vi "App - analyze RUS V6.vi"() -> ()   [LabVIEW 2021] (continued)
 "lorentzian"={"A (VHz)"=0.0, "ω (Hz)"=0.0, "Γ (Hz)"=0.0, "φ (rad)"=0.0, "Q"=0.0, "Norm  Ampl"=0.0, "z∞ (V)"=0.0+0.0i, "4corners"={"z (-pi/2)"=0.0+0.0i, "z(inf)"=0.0+0.0i, "z (pi/2)"=0.0+0.0i, "z center"=0.0+0.0i, "z(0)"=0.0+0.0i, "radius"=0.0}}, "timestamp(min)"=1596.8000000044703, "timestamp"=timestamp(3493823629 s since 1904-01-01), "Magn Field(T)"=0.0}, {"temperature"=41.326, "lorentzian"={"A (VHz)"=0.0, "ω (Hz)"=0.0, "Γ (Hz)"=0.0, "φ (rad)"=0.0, "Q"=0.0, "Norm  Ampl"=0.0, "z∞ (V)"=0.0+0.0i, "4corners"={"z (-pi/2)"=0.0+0.0i, "z(inf)"=0.0+0.0i, "z (pi/2)"=0.0+0.0i, "z center"=0.0+0.0i, "z(0)"=0.0+0.0i, "radius"=0.0}}, "timestamp(min)"=1598.1166666671634, "timestamp"=timestamp(3493823708 s since 1904-01-01), "Magn Field(T)"=0.0}, {"temperature"=41.255, "lorentzian"={"A (VHz)"=0.0, "ω (Hz)"=0.0, "Γ (Hz)"=0.0, "φ (rad)"=0.0, "Q"=0.0, "Norm  Ampl"=0.0, "z∞ (V)"=0.0+0.0i, "4corners"={"z (-pi/2)"=0.0+0.0i, "z(inf)"=0.0+0.0i, "z (pi/2)"=0.0+0.0i, "z center"=0.0+0.0i, "z(0)"=0.0+0.0i, "radius"=0.0}}, "timestamp(min)"=1599.433333337307, "timestamp"=timestamp(3493823787 s since 1904-01-01), "Magn Field(T)"=0.0}, {"temperature"=41.174, "lorentzian"={"A (VHz)"=0.0, "ω (Hz)"=0.0, "Γ (Hz)"=0.0, "φ (rad)"=0.0, "Q"=0.0, "Norm  Ampl"=0.0, "z∞ (V)"=0.0+0.0i, "4corners"={"z (-pi/2)"=0.0+0.0i, "z(inf)"=0.0+0.0i, "z (pi/2)"=0.0+0.0i, "z center"=0.0+0.0i, "z(0)"=0.0+0.0i, "radius"=0.0}}, "timestamp(min)"=1600.7666666656733, "timestamp"=timestamp(3493823867 s since 1904-01-01), "Magn Field(T)"=0.0}, {"temperature"=41.098, "lorentzian"={"A (VHz)"=0.0, "ω (Hz)"=0.0, "Γ (Hz)"=0.0, "φ (rad)"=0.0, "Q"=0.0, "Norm  Ampl"=0.0, "z∞ (V)"=0.0+0.0i, "4corners"={"z (-pi/2)"=0.0+0.0i, "z(inf)"=0.0+0.0i, "z (pi/2)"=0.0+0.0i, "z center"=0.0+0.0i, "z(0)"=0.0+0.0i, "radius"=0.0}}, "timestamp(min)"=1602.0833333358169, "timestamp"=timestamp(3493823946 s since 1904-01-01), "Magn Field(T)"=0.0}, {"temperature"=41.017, "lorentzian"={"A (VHz)"=0.0, "ω (Hz)"=0.0, "Γ (Hz)"=0.0, "φ (rad)"=0.0, "Q"=0.0, "Norm  Ampl"=0.0, "z∞ (V)"=0.0+0.0i, "4corners"={"z (-pi/2)"=0.0+0.0i, "z(inf)"=0.0+0.0i, "z (pi/2)"=0.0+0.0i, "z center"=0.0+0.0i, "z(0)"=0.0+0.0i, "radius"=0.0}}, "timestamp(min)"=1603.3999999985099, "timestamp"=timestamp(3493824025 s since 1904-01-01), "Magn Field(T)"=0.0}, {"temperature"=40.94, "lorentzian"={"A (VHz)"=0.0, "ω (Hz)"=0.0, "Γ (Hz)"=0.0, "φ (rad)"=0.0, "Q"=0.0, "Norm  Ampl"=0.0, "z∞ (V)"=0.0+0.0i, "4corners"={"z (-pi/2)"=0.0+0.0i, "z(inf)"=0.0+0.0i, "z (pi/2)"=0.0+0.0i, "z center"=0.0+0.0i, "z(0)"=0.0+0.0i, "radius"=0.0}}, "timestamp(min)"=1604.7333333343267, "timestamp"=timestamp(3493824105 s since 1904-01-01), "Magn Field(T)"=0.0}, {"temperature"=40.861, "lorentzian"={"A (VHz)"=0.0, "ω (Hz)"=0.0, "Γ (Hz)"=0.0, "φ (rad)"=0.0, "Q"=0.0, "Norm  Ampl"=0.0, "z∞ (V)"=0.0+0.0i, "4corners"={"z (-pi/2)"=0.0+0.0i, "z(inf)"=0.0+0.0i, "z (pi/2)"=0.0+0.0i, "z center"=0.0+0.0i, "z(0)"=0.0+0.0i, "radius"=0.0}}, "timestamp(min)"=1606.0500000044703, "timestamp"=timestamp(3493824184 s since 1904-01-01), "Magn Field(T)"=0.0}, {"temperature"=40.779, "lorentzian"={"A (VHz)"=0.0, "ω (Hz)"=0.0, "Γ (Hz)"=0.0, "φ (rad)"=0.0, "Q"=0.0, "Norm  Ampl"=0.0, "z∞ (V)"=0.0+0.0i, "4corners"={"z (-pi/2)"=0.0+0.0i, "z(inf)"=0.0+0.0i, "z (pi/2)"=0.0+0.0i, "z center"=0.0+0.0i, "z(0)"=0.0+0.0i, "radius"=0.0}}, "timestamp(min)"=1607.3833333328366, "timestamp"=timestamp(3493824264 s since 1904-01-01), "Magn Field(T)"=0.0}, {"temperature"=40.702, "lorentzian"={"A (VHz)"=0.0, "ω (Hz)"=0.0, "Γ (Hz)"=0.0, "φ (rad)"=0.0, "Q"=0.0, "Norm  Ampl"=0.0, "z∞ (V)"=0.0+0.0i, "4corners"={"z (-pi/2)"=0.0+0.0i, "z(inf)"=0.0+0.0i, "z (pi/2)"=0.0+0.0i, "z center"=0.0+0.0i, "z(0)"=0.0+0.0i, "radius"=0.0}}, "timestamp(min)"=1608.7000000029802, "timestamp"=timestamp(3493824343 s since 1904-01-01), "Magn Field(T)"=0.0}, {"temperature"=40.621, "lorentzian"={"A (VHz)"=0.0, "ω (Hz)"=0.0, "Γ (Hz)"=0.0, "φ (rad)"=0.0, "Q"=0.0, "Norm  Ampl"=0.0, "z∞ (V)"=0.0+0.0i, "4corners"={"z (-pi/2)"=0.0+0.0i, "z(inf)"=0.0+0.0i, "z (pi/2)"=0.0+0.0i, "z center"=0.0+0.0i, "z(0)"=0.0+0.0i, "radius"=0.0}}, "timestamp(min)"=1610.0333333313465, "timestamp"=timestamp(3493824423 s since 1904-01-01), "Magn Field(T)"=0.0}, {"temperature"=40.542, "lorentzian"={"A (VHz)"=0.0, "ω (Hz)"=0.0, "Γ (Hz)"=0.0, "φ (rad)"=0.0, "Q"=0.0, "Norm  Ampl"=0.0, "z∞ (V)"=0.0+0.0i, "4corners"={"z (-pi/2)"=0.0+0.0i, "z(inf)"=0.0+0.0i, "z (pi/2)"=0.0+0.0i, "z center"=0.0+0.0i, "z(0)"=0.0+0.0i, "radius"=0.0}}, "timestamp(min)"=1611.3500000014901, "timestamp"=timestamp(3493824502 s since 1904-01-01), "Magn Field(T)"=0.0}, {"temperature"=40.463, "lorentzian"={"A (VHz)"=0.0, "ω (Hz)"=0.0, "Γ (Hz)"=0.0, "φ (rad)"=0.0, "Q"=0.0, "Norm  Ampl"=0.0, "z∞ (V)"=0.0+0.0i, "4corners"={"z (-pi/2)"=0.0+0.0i, "z(inf)"=0.0+0.0i, "z (pi/2)"=0.0+0.0i, "z center"=0.0+0.0i, "z(0)"=0.0+0.0i, "radius"=0.0}}, "timestamp(min)"=1612.683333337307, "timestamp"=timestamp(3493824582 s since 1904-01-01), "Magn Field(T)"=0.0}, {"temperature"=40.383, "lorentzian"={"A (VHz)"=0.0, "ω (Hz)"=0.0, "Γ (Hz)"=0.0, "φ (rad)"=0.0, "Q"=0.0, "Norm  Ampl"=0.0, "z∞ (V)"=0.0+0.0i, "4corners"={"z (-pi/2)"=0.0+0.0i, "z(inf)"=0.0+0.0i, "z (pi/2)"=0.0+0.0i, "z center"=0.0+0.0i, "z(0)"=0.0+0.0i, "radius"=0.0}}, "timestamp(min)"=1614.0, "timestamp"=timestamp(3493824661 s since 1904-01-01), "Magn Field(T)"=0.0}, {"temperature"=40.311, "lorentzian"={"A (VHz)"=0.0, "ω (Hz)"=0.0, "Γ (Hz)"=0.0, "φ (rad)"=0.0, "Q"=0.0, "Norm  Ampl"=0.0, "z∞ (V)"=0.0+0.0i, "4corners"={"z (-pi/2)"=0.0+0.0i, "z(inf)"=0.0+0.0i, "z (pi/2)"=0.0+0.0i, "z center"=0.0+0.0i, "z(0)"=0.0+0.0i, "radius"=0.0}}, "timestamp(min)"=1615.3333333358169, "timestamp"=timestamp(3493824741 s since 1904-01-01), "Magn Field(T)"=0.0}, {"temperature"=40.223, "lorentzian"={"A (VHz)"=0.0, "ω (Hz)"=0.0, "Γ (Hz)"=0.0, "φ (rad)"=0.0, "Q"=0.0, "Norm  Ampl"=0.0, "z∞ (V)"=0.0+0.0i, "4corners"={"z (-pi/2)"=0.0+0.0i, "z(inf)"=0.0+0.0i, "z (pi/2)"=0.0+0.0i, "z center"=0.0+0.0i, "z(0)"=0.0+0.0i, "radius"=0.0}}, "timestamp(min)"=1616.6499999985099, "timestamp"=timestamp(3493824820 s since 1904-01-01), "Magn Field(T)"=0.0}, {"temperature"=40.145, "lorentzian"={"A (VHz)"=0.0, "ω (Hz)"=0.0, "Γ (Hz)"=0.0, "φ (rad)"=0.0, "Q"=0.0, "Norm  Ampl"=0.0, "z∞ (V)"=0.0+0.0i, "4corners"={"z (-pi/2)"=0.0+0.0i, "z(inf)"=0.0+0.0i, "z (pi/2)"=0.0+0.0i, "z center"=0.0+0.0i, "z(0)"=0.0+0.0i, "radius"=0.0}}, "timestamp(min)"=1617.9666666686535, "timestamp"=timestamp(3493824899 s since 1904-01-01), "Magn Field(T)"=0.0}, {"temperature"=40.07, "lorentzian"={"A (VHz)"=0.0, "ω (Hz)"=0.0, "Γ (Hz)"=0.0, "φ (rad)"=0.0, "Q"=0.0, "Norm  Ampl"=0.0, "z∞ (V)"=0.0+0.0i, "4corners"={"z (-pi/2)"=0.0+0.0i, "z(inf)"=0.0+0.0i, "z (pi/2)"=0.0+0.0i, "z center"=0.0+0.0i, "z(0)"=0.0+0.0i, "radius"=0.0}}, "timestamp(min)"=1619.3000000044703, "timestamp"=timestamp(3493824979 s since 1904-01-01), "Magn Field(T)"=0.0}, {"temperature"=39.984, "lorentzian"={"A (VHz)"=0.0, "ω (Hz)"=0.0, "Γ (Hz)"=0.0, "φ (rad)"=0.0, "Q"=0.0, "Norm  Ampl"=0.0, "z∞ (V)"=0.0+0.0i, "4corners"={"z (-pi/2)"=0.0+0.0i, "z(inf)"=0.0+0.0i, "z (pi/2)"=0.0+0.0i, "z center"=0.0+0.0i, "z(0)"=0.0+0.0i, "radius"=0.0}}, "timestamp(min)"=1620.6166666671634, "timestamp"=timestamp(3493825058 s since 1904-01-01), "Magn Field(T)"=0.0}, {"temperature"=39.905, "lorentzian"={"A (VHz)"=0.0, "ω (Hz)"=0.0, "Γ (Hz)"=0.0, "φ (rad)"=0.0, "Q"=0.0, "Norm  Ampl"=0.0, "z∞ (V)"=0.0+0.0i, "4corners"={"z (-pi/2)"=0.0+0.0i, "z(inf)"=0.0+0.0i, "z (pi/2)"=0.0+0.0i, "z center"=0.0+0.0i, "z(0)"=0.0+0.0i, "radius"=0.0}}, "timestamp(min)"=1621.9500000029802, "timestamp"=timestamp(3493825138 s since 1904-01-01), "Magn Field(T)"=0.0}, {"temperature"=39.827, "lorentzian"={"A (VHz)"=0.0, "ω (Hz)"=0.0, "Γ (Hz)"=0.0, "φ (rad)"=0.0, "Q"=0.0, "Norm  Ampl"=0.0, "z∞ (V)"=0.0+0.0i, "4corners"={"z (-pi/2)"=0.0+0.0i, "z(inf)"=0.0+0.0i, "z (pi/2)"=0.0+0.0i, "z center"=0.0+0.0i, "z(0)"=0.0+0.0i, "radius"=0.0}}, "timestamp(min)"=1623.2666666656733, "timestamp"=timestamp(3493825217 s since 1904-01-01), "Magn Field(T)"=0.0}, {"temperature"=39.744, "lorentzian"={"A (VHz)"=0.0, "ω (Hz)"=0.0, "Γ (Hz)"=0.0, "φ (rad)"=0.0, "Q"=0.0, "Norm  Ampl"=0.0, "z∞ (V)"=0.0+0.0i, "4corners"={"z (-pi/2)"=0.0+0.0i, "z(inf)"=0.0+0.0i, "z (pi/2)"=0.0+0.0i, "z center"=0.0+0.0i, "z(0)"=0.0+0.0i, "radius"=0.0}}, "timestamp(min)"=1624.5833333358169, "timestamp"=timestamp(3493825296 s since 1904-01-01), "Magn Field(T)"=0.0}, {"temperature"=39.665, "lorentzian"={"A (VHz)"=0.0, "ω (Hz)"=0.0, "Γ (Hz)"=0.0, "φ (rad)"=0.0, "Q"=0.0, "Norm  Ampl"=0.0, "z∞ (V)"=0.0+0.0i, "4corners"={"z (-pi/2)"=0.0+0.0i, "z(inf)"=0.0+0.0i, "z (pi/2)"=0.0+0.0i, "z center"=0.0+0.0i, "z(0)"=0.0+0.0i, "radius"=0.0}}, "timestamp(min)"=1625.9166666641831, "timestamp"=timestamp(3493825376 s since 1904-01-01), "Magn Field(T)"=0.0}, {"temperature"=39.59, "lorentzian"={"A (VHz)"=0.0, "ω (Hz)"=0.0, "Γ (Hz)"=0.0, "φ (rad)"=0.0, "Q"=0.0, "Norm  Ampl"=0.0, "z∞ (V)"=0.0+0.0i, "4corners"={"z (-pi/2)"=0.0+0.0i, "z(inf)"=0.0+0.0i, "z (pi/2)"=0.0+0.0i, "z center"=0.0+0.0i, "z(0)"=0.0+0.0i, "radius"=0.0}}, "timestamp(min)"=1627.2333333343267, "timestamp"=timestamp(3493825455 s since 1904-01-01), "Magn Field(T)"=0.0}, {"temperature"=39.502, "lorentzian"={"A (VHz)"=0.0, "ω (Hz)"=0.0, "Γ (Hz)"=0.0, "φ (rad)"=0.0, "Q"=0.0, "Norm  Ampl"=0.0, "z∞ (V)"=0.0+0.0i, "4corners"={"z (-pi/2)"=0.0+0.0i, "z(inf)"=0.0+0.0i, "z (pi/2)"=0.0+0.0i, "z center"=0.0+0.0i, "z(0)"=0.0+0.0i, "radius"=0.0}}, "timestamp(min)"=1628.5666666701436, "timestamp"=timestamp(3493825535 s since 1904-01-01), "Magn Field(T)"=0.0}, {"temperature"=39.427, "lorentzian"={"A (VHz)"=0.0, "ω (Hz)"=0.0, "Γ (Hz)"=0.0, "φ (rad)"=0.0, "Q"=0.0, "Norm  Ampl"=0.0, "z∞ (V)"=0.0+0.0i, "4corners"={"z (-pi/2)"=0.0+0.0i, "z(inf)"=0.0+0.0i, "z (pi/2)"=0.0+0.0i, "z center"=0.0+0.0i, "z(0)"=0.0+0.0i, "radius"=0.0}}, "timestamp(min)"=1629.8833333328366, "timestamp"=timestamp(3493825614 s since 1904-01-01), "Magn Field(T)"=0.0}, {"temperature"=39.345, "lorentzian"={"A (VHz)"=0.0, "ω (Hz)"=0.0, "Γ (Hz)"=0.0, "φ (rad)"=0.0, "Q"=0.0, "Norm  Ampl"=0.0, "z∞ (V)"=0.0+0.0i, "4corners"={"z (-pi/2)"=0.0+0.0i, "z(inf)"=0.0+0.0i, "z (pi/2)"=0.0+0.0i, "z center"=0.0+0.0i, "z(0)"=0.0+0.0i, "radius"=0.0}}, "timestamp(min)"=1631.2000000029802, "timestamp"=timestamp(3493825693 s since 1904-01-01), "Magn Field(T)"=0.0}, {"temperature"=39.266, "lorentzian"={"A (VHz)"=0.0, "ω (Hz)"=0.0, "Γ (Hz)"=0.0, "φ (rad)"=0.0, "Q"=0.0, "Norm  Ampl"=0.0, "z∞ (V)"=0.0+0.0i, "4corners"={"z (-pi/2)"=0.0+0.0i, "z(inf)"=0.0+0.0i, "z (pi/2)"=0.0+0.0i, "z center"=0.0+0.0i, "z(0)"=0.0+0.0i, "radius"=0.0}}, "timestamp(min)"=1632.5333333313465, "timestamp"=timestamp(3493825773 s since 1904-01-01), "Magn Field(T)"=0.0}, {"temperature"=39.182, "lorentzian"={"A (VHz)"=0.0, "ω (Hz)"=0.0, "Γ (Hz)"=0.0, "φ (rad)"=0.0, "Q"=0.0, "Norm  Ampl"=0.0, "z∞ (V)"=0.0+0.0i, "4corners"={"z (-pi/2)"=0.0+0.0i, "z(inf)"=0.0+0.0i, "z (pi/2)"=0.0+0.0i, "z center"=0.0+0.0i, "z(0)"=0.0+0.0i, "radius"=0.0}}, "timestamp(min)"=1633.8500000014901, "timestamp"=timestamp(3493825852 s since 1904-01-01), "Magn Field(T)"=0.0}, {"temperature"=39.106, "lorentzian"={"A (VHz)"=0.0, "ω (Hz)"=0.0, "Γ (Hz)"=0.0, "φ (rad)"=0.0, "Q"=0.0, "Norm  Ampl"=0.0, "z∞ (V)"=0.0+0.0i, "4corners"={"z (-pi/2)"=0.0+0.0i, "z(inf)"=0.0+0.0i, "z (pi/2)"=0.0+0.0i, "z center"=0.0+0.0i, "z(0)"=0.0+0.0i, "radius"=0.0}}, "timestamp(min)"=1635.1666666641831, "timestamp"=timestamp(3493825931 s since 1904-01-01), "Magn Field(T)"=0.0}, {"temperature"=39.022, "lorentzian"={"A (VHz)"=0.0, "ω (Hz)"=0.0, "Γ (Hz)"=0.0, "φ (rad)"=0.0, "Q"=0.0, "Norm  Ampl"=0.0, "z∞ (V)"=0.0+0.0i, "4corners"={"z (-pi/2)"=0.0+0.0i, "z(inf)"=0.0+0.0i, "z (pi/2)"=0.0+0.0i, "z center"=0.0+0.0i, "z(0)"=0.0+0.0i, "radius"=0.0}}, "timestamp(min)"=1636.5, "timestamp"=timestamp(3493826011 s since 1904-01-01), "Magn Field(T)"=0.0}, {"temperature"=38.943, "lorentzian"={"A (VHz)"=0.0, "ω (Hz)"=0.0, "Γ (Hz)"=0.0, "φ (rad)"=0.0, "Q"=0.0, "Norm  Ampl"=0.0, "z∞ (V)"=0.0+0.0i, "4corners"={"z (-pi/2)"=0.0+0.0i, "z(inf)"=0.0+0.0i, "z (pi/2)"=0.0+0.0i, "z center"=0.0+0.0i, "z(0)"=0.0+0.0i, "radius"=0.0}}, "timestamp(min)"=1637.8166666701436, "timestamp"=timestamp(3493826090 s since 1904-01-01), "Magn Field(T)"=0.0}, {"temperature"=38.864, "lorentzian"={"A (VHz)"=0.0, "ω (Hz)"=0.0, "Γ (Hz)"=0.0, "φ (rad)"=0.0, "Q"=0.0, "Norm  Ampl"=0.0, "z∞ (V)"=0.0+0.0i, "4corners"={"z (-pi/2)"=0.0+0.0i, "z(inf)"=0.0+0.0i, "z (pi/2)"=0.0+0.0i, "z center"=0.0+0.0i, "z(0)"=0.0+0.0i, "radius"=0.0}}, "timestamp(min)"=1639.1499999985099, "timestamp"=timestamp(3493826170 s since 1904-01-01), "Magn Field(T)"=0.0}, {"temperature"=38.78, "lorentzian"={"A (VHz)"=0.0, "ω (Hz)"=0.0, "Γ (Hz)"=0.0, "φ (rad)"=0.0, "Q"=0.0, "Norm  Ampl"=0.0, "z∞ (V)"=0.0+0.0i, "4corners"={"z (-pi/2)"=0.0+0.0i, "z(inf)"=0.0+0.0i, "z (pi/2)"=0.0+0.0i, "z center"=0.0+0.0i, "z(0)"=0.0+0.0i, "radius"=0.0}}, "timestamp(min)"=1640.4666666686535, "timestamp"=timestamp(3493826249 s since 1904-01-01), "Magn Field(T)"=0.0}, {"temperature"=38.695, "lorentzian"={"A (VHz)"=0.0, "ω (Hz)"=0.0, "Γ (Hz)"=0.0, "φ (rad)"=0.0, "Q"=0.0, "Norm  Ampl"=0.0, "z∞ (V)"=0.0+0.0i, "4corners"={"z (-pi/2)"=0.0+0.0i, "z(inf)"=0.0+0.0i, "z (pi/2)"=0.0+0.0i, "z center"=0.0+0.0i, "z(0)"=0.0+0.0i, "radius"=0.0}}, "timestamp(min)"=1641.8000000044703, "timestamp"=timestamp(3493826329 s since 1904-01-01), "Magn Field(T)"=0.0}, {"temperature"=38.618, "lorentzian"={"A (VHz)"=0.0, "ω (Hz)"=0.0, "Γ (Hz)"=0.0, "φ (rad)"=0.0, "Q"=0.0, "Norm  Ampl"=0.0, "z∞ (V)"=0.0+0.0i, "4corners"={"z (-pi/2)"=0.0+0.0i, "z(inf)"=0.0+0.0i, "z (pi/2)"=0.0+0.0i, "z center"=0.0+0.0i, "z(0)"=0.0+0.0i, "radius"=0.0}}, "timestamp(min)"=1643.1166666671634, "timestamp"=timestamp(3493826408 s since 1904-01-01), "Magn Field(T)"=0.0}, {"temperature"=38.531, "lorentzian"={"A (VHz)"=0.0, "ω (Hz)"=0.0, "Γ (Hz)"=0.0, "φ (rad)"=0.0, "Q"=0.0, "Norm  Ampl"=0.0, "z∞ (V)"=0.0+0.0i, "4corners"={"z (-pi/2)"=0.0+0.0i, "z(inf)"=0.0+0.0i, "z (pi/2)"=0.0+0.0i, "z center"=0.0+0.0i, "z(0)"=0.0+0.0i, "radius"=0.0}}, "timestamp(min)"=1644.433333337307, "timestamp"=timestamp(3493826487 s since 1904-01-01), "Magn Field(T)"=0.0}, {"temperature"=38.455, "lorentzian"={"A (VHz)"=0.0, "ω (Hz)"=0.0, "Γ (Hz)"=0.0, "φ (rad)"=0.0, "Q"=0.0, "Norm  Ampl"=0.0, "z∞ (V)"=0.0+0.0i, "4corners"={"z (-pi/2)"=0.0+0.0i, "z(inf)"=0.0+0.0i, "z (pi/2)"=0.0+0.0i, "z center"=0.0+0.0i, "z(0)"=0.0+0.0i, "radius"=0.0}}, "timestamp(min)"=1645.7666666656733, "timestamp"=timestamp(3493826567 s since 1904-01-01), "Magn Field(T)"=0.0}, {"temperature"=38.37, "lorentzian"={"A (VHz)"=0.0, "ω (Hz)"=0.0, "Γ (Hz)"=0.0, "φ (rad)"=0.0, "Q"=0.0, "Norm  Ampl"=0.0, "z∞ (V)"=0.0+0.0i, "4corners"={"z (-pi/2)"=0.0+0.0i, "z(inf)"=0.0+0.0i, "z (pi/2)"=0.0+0.0i, "z center"=0.0+0.0i, "z(0)"=0.0+0.0i, "radius"=0.0}}, "timestamp(min)"=1647.0833333358169, "timestamp"=timestamp(3493826646 s since 1904-01-01), "Magn Field(T)"=0.0}, {"temperature"=38.286, "lorentzian"={"A (VHz)"=0.0, "ω (Hz)"=0.0, "Γ (Hz)"=0.0, "φ (rad)"=0.0, "Q"=0.0, "Norm  Ampl"=0.0, "z∞ (V)"=0.0+0.0i, "4corners"={"z (-pi/2)"=0.0+0.0i, "z(inf)"=0.0+0.0i, "z (pi/2)"=0.0+0.0i, "z center"=0.0+0.0i, "z(0)"=0.0+0.0i, "radius"=0.0}}, "timestamp(min)"=1648.3999999985099, "timestamp"=timestamp(3493826725 s since 1904-01-01), "Magn Field(T)"=0.0}, {"temperature"=38.203, "lorentzian"={"A (VHz)"=0.0, "ω (Hz)"=0.0, "Γ (Hz)"=0.0, "φ (rad)"=0.0, "Q"=0.0, "Norm  Ampl"=0.0, "z∞ (V)"=0.0+0.0i, "4corners"={"z (-pi/2)"=0.0+0.0i, "z(inf)"=0.0+0.0i, "z (pi/2)"=0.0+0.0i, "z center"=0.0+0.0i, "z(0)"=0.0+0.0i, "radius"=0.0}}, "timestamp(min)"=1649.7333333343267, "timestamp"=timestamp(3493826805 s since 1904-01-01), "Magn Field(T)"=0.0}, {"temperature"=38.122, "lorentzian"={"A (VHz)"=0.0, "ω (Hz)"=0.0, "Γ (Hz)"=0.0, "φ (rad)"=0.0, "Q"=0.0, "Norm  Ampl"=0.0, "z∞ (V)"=0.0+0.0i, "4corners"={"z (-pi/2)"=0.0+0.0i, "z(inf)"=0.0+0.0i, "z (pi/2)"=0.0+0.0i, "z center"=0.0+0.0i, "z(0)"=0.0+0.0i, "radius"=0.0}}, "timestamp(min)"=1651.0500000044703, "timestamp"=timestamp(3493826884 s since 1904-01-01), "Magn Field(T)"=0.0}, {"temperature"=38.042, "lorentzian"={"A (VHz)"=0.0, "ω (Hz)"=0.0, "Γ (Hz)"=0.0, "φ (rad)"=0.0, "Q"=0.0, "Norm  Ampl"=0.0, "z∞ (V)"=0.0+0.0i, "4corners"={"z (-pi/2)"=0.0+0.0i, "z(inf)"=0.0+0.0i, "z (pi/2)"=0.0+0.0i, "z center"=0.0+0.0i, "z(0)"=0.0+0.0i, "radius"=0.0}}, "timestamp(min)"=1652.3833333328366, "timestamp"=timestamp(3493826964 s since 1904-01-01), "Magn Field(T)"=0.0}, {"temperature"=37.958, "lorentzian"={"A (VHz)"=0.0, "ω (Hz)"=0.0, "Γ (Hz)"=0.0, "φ (rad)"=0.0, "Q"=0.0, "Norm  Ampl"=0.0, "z∞ (V)"=0.0+0.0i, "4corners"={"z (-pi/2)"=0.0+0.0i, "z(inf)"=0.0+0.0i, "z (pi/2)"=0.0+0.0i, "z center"=0.0+0.0i, "z(0)"=0.0+0.0i, "radius"=0.0}}, "timestamp(min)"=1653.7000000029802, "timestamp"=timestamp(3493827043 s since 1904-01-01), "Magn Field(T)"=0.0}, {"temperature"=37.876, "lorentzian"={"A (VHz)"=0.0, "ω (Hz)"=0.0, "Γ (Hz)"=0.0, "φ (rad)"=0.0, "Q"=0.0, "Norm  Ampl"=0.0, "z∞ (V)"=0.0+0.0i, "4corners"={"z (-pi/2)"=0.0+0.0i, "z(inf)"=0.0+0.0i, "z (pi/2)"=0.0+0.0i, "z center"=0.0+0.0i, "z(0)"=0.0+0.0i, "radius"=0.0}}, "timestamp(min)"=1655.0166666656733, "timestamp"=timestamp(3493827122 s since 1904-01-01), "Magn Field(T)"=0.0}, {"temperature"=37.797, "lorentzian"={"A (VHz)"=0.0, "ω (Hz)"=0.0, "Γ (Hz)"=0.0, "φ (rad)"=0.0, "Q"=0.0, "Norm  Ampl"=0.0, "z∞ (V)"=0.0+0.0i, "4corners"={"z (-pi/2)"=0.0+0.0i, "z(inf)"=0.0+0.0i, "z (pi/2)"=0.0+0.0i, "z center"=0.0+0.0i, "z(0)"=0.0+0.0i, "radius"=0.0}}, "timestamp(min)"=1656.3500000014901, "timestamp"=timestamp(3493827202 s since 1904-01-01), "Magn Field(T)"=0.0}, {"temperature"=37.711, "lorentzian"={"A (VHz)"=0.0, "ω (Hz)"=0.0, "Γ (Hz)"=0.0, "φ (rad)"=0.0, "Q"=0.0, "Norm  Ampl"=0.0, "z∞ (V)"=0.0+0.0i, "4corners"={"z (-pi/2)"=0.0+0.0i, "z(inf)"=0.0+0.0i, "z (pi/2)"=0.0+0.0i, "z center"=0.0+0.0i, "z(0)"=0.0+0.0i, "radius"=0.0}}, "timestamp(min)"=1657.6666666641831, "timestamp"=timestamp(3493827281 s since 1904-01-01), "Magn Field(T)"=0.0}, {"temperature"=37.627, "lorentzian"={"A (VHz)"=0.0, "ω (Hz)"=0.0, "Γ (Hz)"=0.0, "φ (rad)"=0.0, "Q"=0.0, "Norm  Ampl"=0.0, "z∞ (V)"=0.0+0.0i, "4corners"={"z (-pi/2)"=0.0+0.0i, "z(inf)"=0.0+0.0i, "z (pi/2)"=0.0+0.0i, "z center"=0.0+0.0i, "z(0)"=0.0+0.0i, "radius"=0.0}}, "timestamp(min)"=1658.9833333343267, "timestamp"=timestamp(3493827360 s since 1904-01-01), "Magn Field(T)"=0.0}, {"temperature"=37.544, "lorentzian"={"A (VHz)"=0.0, "ω (Hz)"=0.0, "Γ (Hz)"=0.0, "φ (rad)"=0.0, "Q"=0.0, "Norm  Ampl"=0.0, "z∞ (V)"=0.0+0.0i, "4corners"={"z (-pi/2)"=0.0+0.0i, "z(inf)"=0.0+0.0i, "z (pi/2)"=0.0+0.0i, "z center"=0.0+0.0i, "z(0)"=0.0+0.0i, "radius"=0.0}}, "timestamp(min)"=1660.3166666701436, "timestamp"=timestamp(3493827440 s since 1904-01-01), "Magn Field(T)"=0.0}, {"temperature"=37.459, "lorentzian"={"A (VHz)"=0.0, "ω (Hz)"=0.0, "Γ (Hz)"=0.0, "φ (rad)"=0.0, "Q"=0.0, "Norm  Ampl"=0.0, "z∞ (V)"=0.0+0.0i, "4corners"={"z (-pi/2)"=0.0+0.0i, "z(inf)"=0.0+0.0i, "z (pi/2)"=0.0+0.0i, "z center"=0.0+0.0i, "z(0)"=0.0+0.0i, "radius"=0.0}}, "timestamp(min)"=1661.6333333328366, "timestamp"=timestamp(3493827519 s since 1904-01-01), "Magn Field(T)"=0.0}, {"temperature"=37.378, "lorentzian"={"A (VHz)"=0.0, "ω (Hz)"=0.0, "Γ (Hz)"=0.0, "φ (rad)"=0.0, "Q"=0.0, "Norm  Ampl"=0.0, "z∞ (V)"=0.0+0.0i, "4corners"={"z (-pi/2)"=0.0+0.0i, "z(inf)"=0.0+0.0i, "z (pi/2)"=0.0+0.0i, "z center"=0.0+0.0i, "z(0)"=0.0+0.0i, "radius"=0.0}}, "timestamp(min)"=1662.9666666686535, "timestamp"=timestamp(3493827599 s since 1904-01-01), "Magn Field(T)"=0.0}, {"temperature"=37.297, "lorentzian"={"A (VHz)"=0.0, "ω (Hz)"=0.0, "Γ (Hz)"=0.0, "φ (rad)"=0.0, "Q"=0.0, "Norm  Ampl"=0.0, "z∞ (V)"=0.0+0.0i, "4corners"={"z (-pi/2)"=0.0+0.0i, "z(inf)"=0.0+0.0i, "z (pi/2)"=0.0+0.0i, "z center"=0.0+0.0i, "z(0)"=0.0+0.0i, "radius"=0.0}}, "timestamp(min)"=1664.2833333313465, "timestamp"=timestamp(3493827678 s since 1904-01-01), "Magn Field(T)"=0.0}, {"temperature"=37.206, "lorentzian"={"A (VHz)"=0.0, "ω (Hz)"=0.0, "Γ (Hz)"=0.0, "φ (rad)"=0.0, "Q"=0.0, "Norm  Ampl"=0.0, "z∞ (V)"=0.0+0.0i, "4corners"={"z (-pi/2)"=0.0+0.0i, "z(inf)"=0.0+0.0i, "z (pi/2)"=0.0+0.0i, "z center"=0.0+0.0i, "z(0)"=0.0+0.0i, "radius"=0.0}}, "timestamp(min)"=1665.6000000014901, "timestamp"=timestamp(3493827757 s since 1904-01-01), "Magn Field(T)"=0.0}, {"temperature"=37.129, "lorentzian"={"A (VHz)"=0.0, "ω (Hz)"=0.0, "Γ (Hz)"=0.0, "φ (rad)"=0.0, "Q"=0.0, "Norm  Ampl"=0.0, "z∞ (V)"=0.0+0.0i, "4corners"={"z (-pi/2)"=0.0+0.0i, "z(inf)"=0.0+0.0i, "z (pi/2)"=0.0+0.0i, "z center"=0.0+0.0i, "z(0)"=0.0+0.0i, "radius"=0.0}}, "timestamp(min)"=1666.933333337307, "timestamp"=timestamp(3493827837 s since 1904-01-01), "Magn Field(T)"=0.0}, {"temperature"=37.038, "lorentzian"={"A (VHz)"=0.0, "ω (Hz)"=0.0, "Γ (Hz)"=0.0, "φ (rad)"=0.0, "Q"=0.0, "Norm  Ampl"=0.0, "z∞ (V)"=0.0+0.0i, "4corners"={"z (-pi/2)"=0.0+0.0i, "z(inf)"=0.0+0.0i, "z (pi/2)"=0.0+0.0i, "z center"=0.0+0.0i, "z(0)"=0.0+0.0i, "radius"=0.0}}, "timestamp(min)"=1668.25, "timestamp"=timestamp(3493827916 s since 1904-01-01), "Magn Field(T)"=0.0}, {"temperature"=36.964, "lorentzian"={"A (VHz)"=0.0, "ω (Hz)"=0.0, "Γ (Hz)"=0.0, "φ (rad)"=0.0, "Q"=0.0, "Norm  Ampl"=0.0, "z∞ (V)"=0.0+0.0i, "4corners"={"z (-pi/2)"=0.0+0.0i, "z(inf)"=0.0+0.0i, "z (pi/2)"=0.0+0.0i, "z center"=0.0+0.0i, "z(0)"=0.0+0.0i, "radius"=0.0}}, "timestamp(min)"=1669.5666666701436, "timestamp"=timestamp(3493827995 s since 1904-01-01), "Magn Field(T)"=0.0}, {"temperature"=36.875, "lorentzian"={"A (VHz)"=0.0, "ω (Hz)"=0.0, "Γ (Hz)"=0.0, "φ (rad)"=0.0, "Q"=0.0, "Norm  Ampl"=0.0, "z∞ (V)"=0.0+0.0i, "4corners"={"z (-pi/2)"=0.0+0.0i, "z(inf)"=0.0+0.0i, "z (pi/2)"=0.0+0.0i, "z center"=0.0+0.0i, "z(0)"=0.0+0.0i, "radius"=0.0}}, "timestamp(min)"=1670.8999999985099, "timestamp"=timestamp(3493828075 s since 1904-01-01), "Magn Field(T)"=0.0}, {"temperature"=36.787, "lorentzian"={"A (VHz)"=0.0, "ω (Hz)"=0.0, "Γ (Hz)"=0.0, "φ (rad)"=0.0, "Q"=0.0, "Norm  Ampl"=0.0, "z∞ (V)"=0.0+0.0i, "4corners"={"z (-pi/2)"=0.0+0.0i, "z(inf)"=0.0+0.0i, "z (pi/2)"=0.0+0.0i, "z center"=0.0+0.0i, "z(0)"=0.0+0.0i, "radius"=0.0}}, "timestamp(min)"=1672.2166666686535, "timestamp"=timestamp(3493828154 s since 1904-01-01), "Magn Field(T)"=0.0}, {"temperature"=36.71, "lorentzian"={"A (VHz)"=0.0, "ω (Hz)"=0.0, "Γ (Hz)"=0.0, "φ (rad)"=0.0, "Q"=0.0, "Norm  Ampl"=0.0, "z∞ (V)"=0.0+0.0i, "4corners"={"z (-pi/2)"=0.0+0.0i, "z(inf)"=0.0+0.0i, "z (pi/2)"=0.0+0.0i, "z center"=0.0+0.0i, "z(0)"=0.0+0.0i, "radius"=0.0}}, "timestamp(min)"=1673.5500000044703, "timestamp"=timestamp(3493828234 s since 1904-01-01), "Magn Field(T)"=0.0}, {"temperature"=36.616, "lorentzian"={"A (VHz)"=0.0, "ω (Hz)"=0.0, "Γ (Hz)"=0.0, "φ (rad)"=0.0, "Q"=0.0, "Norm  Ampl"=0.0, "z∞ (V)"=0.0+0.0i, "4corners"={"z (-pi/2)"=0.0+0.0i, "z(inf)"=0.0+0.0i, "z (pi/2)"=0.0+0.0i, "z center"=0.0+0.0i, "z(0)"=0.0+0.0i, "radius"=0.0}}, "timestamp(min)"=1674.8666666671634, "timestamp"=timestamp(3493828313 s since 1904-01-01), "Magn Field(T)"=0.0}, {"temperature"=36.538, "lorentzian"={"A (VHz)"=0.0, "ω (Hz)"=0.0, "Γ (Hz)"=0.0, "φ (rad)"=0.0, "Q"=0.0, "Norm  Ampl"=0.0, "z∞ (V)"=0.0+0.0i, "4corners"={"z (-pi/2)"=0.0+0.0i, "z(inf)"=0.0+0.0i, "z (pi/2)"=0.0+0.0i, "z center"=0.0+0.0i, "z(0)"=0.0+0.0i, "radius"=0.0}}, "timestamp(min)"=1676.183333337307, "timestamp"=timestamp(3493828392 s since 1904-01-01), "Magn Field(T)"=0.0}, {"temperature"=36.457, "lorentzian"={"A (VHz)"=0.0, "ω (Hz)"=0.0, "Γ (Hz)"=0.0, "φ (rad)"=0.0, "Q"=0.0, "Norm  Ampl"=0.0, "z∞ (V)"=0.0+0.0i, "4corners"={"z (-pi/2)"=0.0+0.0i, "z(inf)"=0.0+0.0i, "z (pi/2)"=0.0+0.0i, "z center"=0.0+0.0i, "z(0)"=0.0+0.0i, "radius"=0.0}}, "timestamp(min)"=1677.5166666656733, "timestamp"=timestamp(3493828472 s since 1904-01-01), "Magn Field(T)"=0.0}, {"temperature"=36.365, "lorentzian"={"A (VHz)"=0.0, "ω (Hz)"=0.0, "Γ (Hz)"=0.0, "φ (rad)"=0.0, "Q"=0.0, "Norm  Ampl"=0.0, "z∞ (V)"=0.0+0.0i, "4corners"={"z (-pi/2)"=0.0+0.0i, "z(inf)"=0.0+0.0i, "z (pi/2)"=0.0+0.0i, "z center"=0.0+0.0i, "z(0)"=0.0+0.0i, "radius"=0.0}}, "timestamp(min)"=1678.8333333358169, "timestamp"=timestamp(3493828551 s since 1904-01-01), "Magn Field(T)"=0.0}, {"temperature"=36.288, "lorentzian"={"A (VHz)"=0.0, "ω (Hz)"=0.0, "Γ (Hz)"=0.0, "φ (rad)"=0.0, "Q"=0.0, "Norm  Ampl"=0.0, "z∞ (V)"=0.0+0.0i, "4corners"={"z (-pi/2)"=0.0+0.0i, "z(inf)"=0.0+0.0i, "z (pi/2)"=0.0+0.0i, "z center"=0.0+0.0i, "z(0)"=0.0+0.0i, "radius"=0.0}}, "timestamp(min)"=1680.1666666641831, "timestamp"=timestamp(3493828631 s since 1904-01-01), "Magn Field(T)"=0.0}, {"temperature"=36.202, "lorentzian"={"A (VHz)"=0.0, "ω (Hz)"=0.0, "Γ (Hz)"=0.0, "φ (rad)"=0.0, "Q"=0.0, "Norm  Ampl"=0.0, "z∞ (V)"=0.0+0.0i, "4corners"={"z (-pi/2)"=0.0+0.0i, "z(inf)"=0.0+0.0i, "z (pi/2)"=0.0+0.0i, "z center"=0.0+0.0i, "z(0)"=0.0+0.0i, "radius"=0.0}}, "timestamp(min)"=1681.4833333343267, "timestamp"=timestamp(3493828710 s since 1904-01-01), "Magn Field(T)"=0.0}, {"temperature"=36.116, "lorentzian"={"A (VHz)"=0.0, "ω (Hz)"=0.0, "Γ (Hz)"=0.0, "φ (rad)"=0.0, "Q"=0.0, "Norm  Ampl"=0.0, "z∞ (V)"=0.0+0.0i, "4corners"={"z (-pi/2)"=0.0+0.0i, "z(inf)"=0.0+0.0i, "z (pi/2)"=0.0+0.0i, "z center"=0.0+0.0i, "z(0)"=0.0+0.0i, "radius"=0.0}}, "timestamp(min)"=1682.8000000044703, "timestamp"=timestamp(3493828789 s since 1904-01-01), "Magn Field(T)"=0.0}, {"temperature"=36.028, "lorentzian"={"A (VHz)"=0.0, "ω (Hz)"=0.0, "Γ (Hz)"=0.0, "φ (rad)"=0.0, "Q"=0.0, "Norm  Ampl"=0.0, "z∞ (V)"=0.0+0.0i, "4corners"={"z (-pi/2)"=0.0+0.0i, "z(inf)"=0.0+0.0i, "z (pi/2)"=0.0+0.0i, "z center"=0.0+0.0i, "z(0)"=0.0+0.0i, "radius"=0.0}}, "timestamp(min)"=1684.1333333328366, "timestamp"=timestamp(3493828869 s since 1904-01-01), "Magn Field(T)"=0.0}, {"temperature"=35.946, "lorentzian"={"A (VHz)"=0.0, "ω (Hz)"=0.0, "Γ (Hz)"=0.0, "φ (rad)"=0.0, "Q"=0.0, "Norm  Ampl"=0.0, "z∞ (V)"=0.0+0.0i, "4corners"={"z (-pi/2)"=0.0+0.0i, "z(inf)"=0.0+0.0i, "z (pi/2)"=0.0+0.0i, "z center"=0.0+0.0i, "z(0)"=0.0+0.0i, "radius"=0.0}}, "timestamp(min)"=1685.4500000029802, "timestamp"=timestamp(3493828948 s since 1904-01-01), "Magn Field(T)"=0.0}, {"temperature"=35.859, "lorentzian"={"A (VHz)"=0.0, "ω (Hz)"=0.0, "Γ (Hz)"=0.0, "φ (rad)"=0.0, "Q"=0.0, "Norm  Ampl"=0.0, "z∞ (V)"=0.0+0.0i, "4corners"={"z (-pi/2)"=0.0+0.0i, "z(inf)"=0.0+0.0i, "z (pi/2)"=0.0+0.0i, "z center"=0.0+0.0i, "z(0)"=0.0+0.0i, "radius"=0.0}}, "timestamp(min)"=1686.7666666656733, "timestamp"=timestamp(3493829027 s since 1904-01-01), "Magn Field(T)"=0.0}, {"temperature"=35.776, "lorentzian"={"A (VHz)"=0.0, "ω (Hz)"=0.0, "Γ (Hz)"=0.0, "φ (rad)"=0.0, "Q"=0.0, "Norm  Ampl"=0.0, "z∞ (V)"=0.0+0.0i, "4corners"={"z (-pi/2)"=0.0+0.0i, "z(inf)"=0.0+0.0i, "z (pi/2)"=0.0+0.0i, "z center"=0.0+0.0i, "z(0)"=0.0+0.0i, "radius"=0.0}}, "timestamp(min)"=1688.1000000014901, "timestamp"=timestamp(3493829107 s since 1904-01-01), "Magn Field(T)"=0.0}, {"temperature"=35.691, "lorentzian"={"A (VHz)"=0.0, "ω (Hz)"=0.0, "Γ (Hz)"=0.0, "φ (rad)"=0.0, "Q"=0.0, "Norm  Ampl"=0.0, "z∞ (V)"=0.0+0.0i, "4corners"={"z (-pi/2)"=0.0+0.0i, "z(inf)"=0.0+0.0i, "z (pi/2)"=0.0+0.0i, "z center"=0.0+0.0i, "z(0)"=0.0+0.0i, "radius"=0.0}}, "timestamp(min)"=1689.4166666641831, "timestamp"=timestamp(3493829186 s since 1904-01-01), "Magn Field(T)"=0.0}, {"temperature"=35.608, "lorentzian"={"A (VHz)"=0.0, "ω (Hz)"=0.0, "Γ (Hz)"=0.0, "φ (rad)"=0.0, "Q"=0.0, "Norm  Ampl"=0.0, "z∞ (V)"=0.0+0.0i, "4corners"={"z (-pi/2)"=0.0+0.0i, "z(inf)"=0.0+0.0i, "z (pi/2)"=0.0+0.0i, "z center"=0.0+0.0i, "z(0)"=0.0+0.0i, "radius"=0.0}}, "timestamp(min)"=1690.75, "timestamp"=timestamp(3493829266 s since 1904-01-01), "Magn Field(T)"=0.0}, {"temperature"=35.519, "lorentzian"={"A (VHz)"=0.0, "ω (Hz)"=0.0, "Γ (Hz)"=0.0, "φ (rad)"=0.0, "Q"=0.0, "Norm  Ampl"=0.0, "z∞ (V)"=0.0+0.0i, "4corners"={"z (-pi/2)"=0.0+0.0i, "z(inf)"=0.0+0.0i, "z (pi/2)"=0.0+0.0i, "z center"=0.0+0.0i, "z(0)"=0.0+0.0i, "radius"=0.0}}, "timestamp(min)"=1692.0666666701436, "timestamp"=timestamp(3493829345 s since 1904-01-01), "Magn Field(T)"=0.0}, {"temperature"=35.437, "lorentzian"={"A (VHz)"=0.0, "ω (Hz)"=0.0, "Γ (Hz)"=0.0, "φ (rad)"=0.0, "Q"=0.0, "Norm  Ampl"=0.0, "z∞ (V)"=0.0+0.0i, "4corners"={"z (-pi/2)"=0.0+0.0i, "z(inf)"=0.0+0.0i, "z (pi/2)"=0.0+0.0i, "z center"=0.0+0.0i, "z(0)"=0.0+0.0i, "radius"=0.0}}, "timestamp(min)"=1693.3833333328366, "timestamp"=timestamp(3493829424 s since 1904-01-01), "Magn Field(T)"=0.0}, {"temperature"=35.349, "lorentzian"={"A (VHz)"=0.0, "ω (Hz)"=0.0, "Γ (Hz)"=0.0, "φ (rad)"=0.0, "Q"=0.0, "Norm  Ampl"=0.0, "z∞ (V)"=0.0+0.0i, "4corners"={"z (-pi/2)"=0.0+0.0i, "z(inf)"=0.0+0.0i, "z (pi/2)"=0.0+0.0i, "z center"=0.0+0.0i, "z(0)"=0.0+0.0i, "radius"=0.0}}, "timestamp(min)"=1694.7166666686535, "timestamp"=timestamp(3493829504 s since 1904-01-01), "Magn Field(T)"=0.0}, {"temperature"=35.264, "lorentzian"={"A (VHz)"=0.0, "ω (Hz)"=0.0, "Γ (Hz)"=0.0, "φ (rad)"=0.0, "Q"=0.0, "Norm  Ampl"=0.0, "z∞ (V)"=0.0+0.0i, "4corners"={"z (-pi/2)"=0.0+0.0i, "z(inf)"=0.0+0.0i, "z (pi/2)"=0.0+0.0i, "z center"=0.0+0.0i, "z(0)"=0.0+0.0i, "radius"=0.0}}, "timestamp(min)"=1696.0333333313465, "timestamp"=timestamp(3493829583 s since 1904-01-01), "Magn Field(T)"=0.0}, {"temperature"=35.178, "lorentzian"={"A (VHz)"=0.0, "ω (Hz)"=0.0, "Γ (Hz)"=0.0, "φ (rad)"=0.0, "Q"=0.0, "Norm  Ampl"=0.0, "z∞ (V)"=0.0+0.0i, "4corners"={"z (-pi/2)"=0.0+0.0i, "z(inf)"=0.0+0.0i, "z (pi/2)"=0.0+0.0i, "z center"=0.0+0.0i, "z(0)"=0.0+0.0i, "radius"=0.0}}, "timestamp(min)"=1697.3666666671634, "timestamp"=timestamp(3493829663 s since 1904-01-01), "Magn Field(T)"=0.0}, {"temperature"=35.091, "lorentzian"={"A (VHz)"=0.0, "ω (Hz)"=0.0, "Γ (Hz)"=0.0, "φ (rad)"=0.0, "Q"=0.0, "Norm  Ampl"=0.0, "z∞ (V)"=0.0+0.0i, "4corners"={"z (-pi/2)"=0.0+0.0i, "z(inf)"=0.0+0.0i, "z (pi/2)"=0.0+0.0i, "z center"=0.0+0.0i, "z(0)"=0.0+0.0i, "radius"=0.0}}, "timestamp(min)"=1698.683333337307, "timestamp"=timestamp(3493829742 s since 1904-01-01), "Magn Field(T)"=0.0}, {"temperature"=35.004, "lorentzian"={"A (VHz)"=0.0, "ω (Hz)"=0.0, "Γ (Hz)"=0.0, "φ (rad)"=0.0, "Q"=0.0, "Norm  Ampl"=0.0, "z∞ (V)"=0.0+0.0i, "4corners"={"z (-pi/2)"=0.0+0.0i, "z(inf)"=0.0+0.0i, "z (pi/2)"=0.0+0.0i, "z center"=0.0+0.0i, "z(0)"=0.0+0.0i, "radius"=0.0}}, "timestamp(min)"=1700.0, "timestamp"=timestamp(3493829821 s since 1904-01-01), "Magn Field(T)"=0.0}, {"temperature"=34.918, "lorentzian"={"A (VHz)"=0.0, "ω (Hz)"=0.0, "Γ (Hz)"=0.0, "φ (rad)"=0.0, "Q"=0.0, "Norm  Ampl"=0.0, "z∞ (V)"=0.0+0.0i, "4corners"={"z (-pi/2)"=0.0+0.0i, "z(inf)"=0.0+0.0i, "z (pi/2)"=0.0+0.0i, "z center"=0.0+0.0i, "z(0)"=0.0+0.0i, "radius"=0.0}}, "timestamp(min)"=1701.3333333358169, "timestamp"=timestamp(3493829901 s since 1904-01-01), "Magn Field(T)"=0.0}, {"temperature"=34.836, "lorentzian"={"A (VHz)"=0.0, "ω (Hz)"=0.0, "Γ (Hz)"=0.0, "φ (rad)"=0.0, "Q"=0.0, "Norm  Ampl"=0.0, "z∞ (V)"=0.0+0.0i, "4corners"={"z (-pi/2)"=0.0+0.0i, "z(inf)"=0.0+0.0i, "z (pi/2)"=0.0+0.0i, "z center"=0.0+0.0i, "z(0)"=0.0+0.0i, "radius"=0.0}}, "timestamp(min)"=1702.6499999985099, "timestamp"=timestamp(3493829980 s since 1904-01-01), "Magn Field(T)"=0.0}, {"temperature"=34.745, "lorentzian"={"A (VHz)"=0.0, "ω (Hz)"=0.0, "Γ (Hz)"=0.0, "φ (rad)"=0.0, "Q"=0.0, "Norm  Ampl"=0.0, "z∞ (V)"=0.0+0.0i, "4corners"={"z (-pi/2)"=0.0+0.0i, "z(inf)"=0.0+0.0i, "z (pi/2)"=0.0+0.0i, "z center"=0.0+0.0i, "z(0)"=0.0+0.0i, "radius"=0.0}}, "timestamp(min)"=1703.9666666686535, "timestamp"=timestamp(3493830059 s since 1904-01-01), "Magn Field(T)"=0.0}, {"temperature"=34.657, "lorentzian"={"A (VHz)"=0.0, "ω (Hz)"=0.0, "Γ (Hz)"=0.0, "φ (rad)"=0.0, "Q"=0.0, "Norm  Ampl"=0.0, "z∞ (V)"=0.0+0.0i, "4corners"={"z (-pi/2)"=0.0+0.0i, "z(inf)"=0.0+0.0i, "z (pi/2)"=0.0+0.0i, "z center"=0.0+0.0i, "z(0)"=0.0+0.0i, "radius"=0.0}}, "timestamp(min)"=1705.3000000044703, "timestamp"=timestamp(3493830139 s since 1904-01-01), "Magn Field(T)"=0.0}, {"temperature"=34.57, "lorentzian"={"A (VHz)"=0.0, "ω (Hz)"=0.0, "Γ (Hz)"=0.0, "φ (rad)"=0.0, "Q"=0.0, "Norm  Ampl"=0.0, "z∞ (V)"=0.0+0.0i, "4corners"={"z (-pi/2)"=0.0+0.0i, "z(inf)"=0.0+0.0i, "z (pi/2)"=0.0+0.0i, "z center"=0.0+0.0i, "z(0)"=0.0+0.0i, "radius"=0.0}}, "timestamp(min)"=1706.6166666671634, "timestamp"=timestamp(3493830218 s since 1904-01-01), "Magn Field(T)"=0.0}, {"temperature"=34.486, "lorentzian"={"A (VHz)"=0.0, "ω (Hz)"=0.0, "Γ (Hz)"=0.0, "φ (rad)"=0.0, "Q"=0.0, "Norm  Ampl"=0.0, "z∞ (V)"=0.0+0.0i, "4corners"={"z (-pi/2)"=0.0+0.0i, "z(inf)"=0.0+0.0i, "z (pi/2)"=0.0+0.0i, "z center"=0.0+0.0i, "z(0)"=0.0+0.0i, "radius"=0.0}}, "timestamp(min)"=1707.9500000029802, "timestamp"=timestamp(3493830298 s since 1904-01-01), "Magn Field(T)"=0.0}, {"temperature"=34.396, "lorentzian"={"A (VHz)"=0.0, "ω (Hz)"=0.0, "Γ (Hz)"=0.0, "φ (rad)"=0.0, "Q"=0.0, "Norm  Ampl"=0.0, "z∞ (V)"=0.0+0.0i, "4corners"={"z (-pi/2)"=0.0+0.0i, "z(inf)"=0.0+0.0i, "z (pi/2)"=0.0+0.0i, "z center"=0.0+0.0i, "z(0)"=0.0+0.0i, "radius"=0.0}}, "timestamp(min)"=1709.2666666656733, "timestamp"=timestamp(3493830377 s since 1904-01-01), "Magn Field(T)"=0.0}, {"temperature"=34.305, "lorentzian"={"A (VHz)"=0.0, "ω (Hz)"=0.0, "Γ (Hz)"=0.0, "φ (rad)"=0.0, "Q"=0.0, "Norm  Ampl"=0.0, "z∞ (V)"=0.0+0.0i, "4corners"={"z (-pi/2)"=0.0+0.0i, "z(inf)"=0.0+0.0i, "z (pi/2)"=0.0+0.0i, "z center"=0.0+0.0i, "z(0)"=0.0+0.0i, "radius"=0.0}}, "timestamp(min)"=1710.5833333358169, "timestamp"=timestamp(3493830456 s since 1904-01-01), "Magn Field(T)"=0.0}, {"temperature"=34.228, "lorentzian"={"A (VHz)"=0.0, "ω (Hz)"=0.0, "Γ (Hz)"=0.0, "φ (rad)"=0.0, "Q"=0.0, "Norm  Ampl"=0.0, "z∞ (V)"=0.0+0.0i, "4corners"={"z (-pi/2)"=0.0+0.0i, "z(inf)"=0.0+0.0i, "z (pi/2)"=0.0+0.0i, "z center"=0.0+0.0i, "z(0)"=0.0+0.0i, "radius"=0.0}}, "timestamp(min)"=1711.9166666641831, "timestamp"=timestamp(3493830536 s since 1904-01-01), "Magn Field(T)"=0.0}, {"temperature"=34.134, "lorentzian"={"A (VHz)"=0.0, "ω (Hz)"=0.0, "Γ (Hz)"=0.0, "φ (rad)"=0.0, "Q"=0.0, "Norm  Ampl"=0.0, "z∞ (V)"=0.0+0.0i, "4corners"={"z (-pi/2)"=0.0+0.0i, "z(inf)"=0.0+0.0i, "z (pi/2)"=0.0+0.0i, "z center"=0.0+0.0i, "z(0)"=0.0+0.0i, "radius"=0.0}}, "timestamp(min)"=1713.2333333343267, "timestamp"=timestamp(3493830615 s since 1904-01-01), "Magn Field(T)"=0.0}, {"temperature"=34.046, "lorentzian"={"A (VHz)"=0.0, "ω (Hz)"=0.0, "Γ (Hz)"=0.0, "φ (rad)"=0.0, "Q"=0.0, "Norm  Ampl"=0.0, "z∞ (V)"=0.0+0.0i, "4corners"={"z (-pi/2)"=0.0+0.0i, "z(inf)"=0.0+0.0i, "z (pi/2)"=0.0+0.0i, "z center"=0.0+0.0i, "z(0)"=0.0+0.0i, "radius"=0.0}}, "timestamp(min)"=1714.5500000044703, "timestamp"=timestamp(3493830694 s since 1904-01-01), "Magn Field(T)"=0.0}, {"temperature"=33.968, "lorentzian"={"A (VHz)"=0.0, "ω (Hz)"=0.0, "Γ (Hz)"=0.0, "φ (rad)"=0.0, "Q"=0.0, "Norm  Ampl"=0.0, "z∞ (V)"=0.0+0.0i, "4corners"={"z (-pi/2)"=0.0+0.0i, "z(inf)"=0.0+0.0i, "z (pi/2)"=0.0+0.0i, "z center"=0.0+0.0i, "z(0)"=0.0+0.0i, "radius"=0.0}}, "timestamp(min)"=1715.8833333328366, "timestamp"=timestamp(3493830774 s since 1904-01-01), "Magn Field(T)"=0.0}, {"temperature"=33.87, "lorentzian"={"A (VHz)"=0.0, "ω (Hz)"=0.0, "Γ (Hz)"=0.0, "φ (rad)"=0.0, "Q"=0.0, "Norm  Ampl"=0.0, "z∞ (V)"=0.0+0.0i, "4corners"={"z (-pi/2)"=0.0+0.0i, "z(inf)"=0.0+0.0i, "z (pi/2)"=0.0+0.0i, "z center"=0.0+0.0i, "z(0)"=0.0+0.0i, "radius"=0.0}}, "timestamp(min)"=1717.2000000029802, "timestamp"=timestamp(3493830853 s since 1904-01-01), "Magn Field(T)"=0.0}, {"temperature"=33.785, "lorentzian"={"A (VHz)"=0.0, "ω (Hz)"=0.0, "Γ (Hz)"=0.0, "φ (rad)"=0.0, "Q"=0.0, "Norm  Ampl"=0.0, "z∞ (V)"=0.0+0.0i, "4corners"={"z (-pi/2)"=0.0+0.0i, "z(inf)"=0.0+0.0i, "z (pi/2)"=0.0+0.0i, "z center"=0.0+0.0i, "z(0)"=0.0+0.0i, "radius"=0.0}}, "timestamp(min)"=1718.5333333313465, "timestamp"=timestamp(3493830933 s since 1904-01-01), "Magn Field(T)"=0.0}, {"temperature"=33.699, "lorentzian"={"A (VHz)"=0.0, "ω (Hz)"=0.0, "Γ (Hz)"=0.0, "φ (rad)"=0.0, "Q"=0.0, "Norm  Ampl"=0.0, "z∞ (V)"=0.0+0.0i, "4corners"={"z (-pi/2)"=0.0+0.0i, "z(inf)"=0.0+0.0i, "z (pi/2)"=0.0+0.0i, "z center"=0.0+0.0i, "z(0)"=0.0+0.0i, "radius"=0.0}}, "timestamp(min)"=1719.8500000014901, "timestamp"=timestamp(3493831012 s since 1904-01-01), "Magn Field(T)"=0.0}, {"temperature"=33.604, "lorentzian"={"A (VHz)"=0.0, "ω (Hz)"=0.0, "Γ (Hz)"=0.0, "φ (rad)"=0.0, "Q"=0.0, "Norm  Ampl"=0.0, "z∞ (V)"=0.0+0.0i, "4corners"={"z (-pi/2)"=0.0+0.0i, "z(inf)"=0.0+0.0i, "z (pi/2)"=0.0+0.0i, "z center"=0.0+0.0i, "z(0)"=0.0+0.0i, "radius"=0.0}}, "timestamp(min)"=1721.1666666641831, "timestamp"=timestamp(3493831091 s since 1904-01-01), "Magn Field(T)"=0.0}, {"temperature"=33.517, "lorentzian"={"A (VHz)"=0.0, "ω (Hz)"=0.0, "Γ (Hz)"=0.0, "φ (rad)"=0.0, "Q"=0.0, "Norm  Ampl"=0.0, "z∞ (V)"=0.0+0.0i, "4corners"={"z (-pi/2)"=0.0+0.0i, "z(inf)"=0.0+0.0i, "z (pi/2)"=0.0+0.0i, "z center"=0.0+0.0i, "z(0)"=0.0+0.0i, "radius"=0.0}}, "timestamp(min)"=1722.5, "timestamp"=timestamp(3493831171 s since 1904-01-01), "Magn Field(T)"=0.0}, {"temperature"=33.438, "lorentzian"={"A (VHz)"=0.0, "ω (Hz)"=0.0, "Γ (Hz)"=0.0, "φ (rad)"=0.0, "Q"=0.0, "Norm  Ampl"=0.0, "z∞ (V)"=0.0+0.0i, "4corners"={"z (-pi/2)"=0.0+0.0i, "z(inf)"=0.0+0.0i, "z (pi/2)"=0.0+0.0i, "z center"=0.0+0.0i, "z(0)"=0.0+0.0i, "radius"=0.0}}, "timestamp(min)"=1723.8166666701436, "timestamp"=timestamp(3493831250 s since 1904-01-01), "Magn Field(T)"=0.0}, {"temperature"=33.342, "lorentzian"={"A (VHz)"=0.0, "ω (Hz)"=0.0, "Γ (Hz)"=0.0, "φ (rad)"=0.0, "Q"=0.0, "Norm  Ampl"=0.0, "z∞ (V)"=0.0+0.0i, "4corners"={"z (-pi/2)"=0.0+0.0i, "z(inf)"=0.0+0.0i, "z (pi/2)"=0.0+0.0i, "z center"=0.0+0.0i, "z(0)"=0.0+0.0i, "radius"=0.0}}, "timestamp(min)"=1725.1499999985099, "timestamp"=timestamp(3493831330 s since 1904-01-01), "Magn Field(T)"=0.0}, {"temperature"=33.262, "lorentzian"={"A (VHz)"=0.0, "ω (Hz)"=0.0, "Γ (Hz)"=0.0, "φ (rad)"=0.0, "Q"=0.0, "Norm  Ampl"=0.0, "z∞ (V)"=0.0+0.0i, "4corners"={"z (-pi/2)"=0.0+0.0i, "z(inf)"=0.0+0.0i, "z (pi/2)"=0.0+0.0i, "z center"=0.0+0.0i, "z(0)"=0.0+0.0i, "radius"=0.0}}, "timestamp(min)"=1726.4666666686535, "timestamp"=timestamp(3493831409 s since 1904-01-01), "Magn Field(T)"=0.0}, {"temperature"=33.17, "lorentzian"={"A (VHz)"=0.0, "ω (Hz)"=0.0, "Γ (Hz)"=0.0, "φ (rad)"=0.0, "Q"=0.0, "Norm  Ampl"=0.0, "z∞ (V)"=0.0+0.0i, "4corners"={"z (-pi/2)"=0.0+0.0i, "z(inf)"=0.0+0.0i, "z (pi/2)"=0.0+0.0i, "z center"=0.0+0.0i, "z(0)"=0.0+0.0i, "radius"=0.0}}, "timestamp(min)"=1727.7833333313465, "timestamp"=timestamp(3493831488 s since 1904-01-01), "Magn Field(T)"=0.0}, {"temperature"=33.079, "lorentzian"={"A (VHz)"=0.0, "ω (Hz)"=0.0, "Γ (Hz)"=0.0, "φ (rad)"=0.0, "Q"=0.0, "Norm  Ampl"=0.0, "z∞ (V)"=0.0+0.0i, "4corners"={"z (-pi/2)"=0.0+0.0i, "z(inf)"=0.0+0.0i, "z (pi/2)"=0.0+0.0i, "z center"=0.0+0.0i, "z(0)"=0.0+0.0i, "radius"=0.0}}, "timestamp(min)"=1729.1166666671634, "timestamp"=timestamp(3493831568 s since 1904-01-01), "Magn Field(T)"=0.0}, {"temperature"=32.992, "lorentzian"={"A (VHz)"=0.0, "ω (Hz)"=0.0, "Γ (Hz)"=0.0, "φ (rad)"=0.0, "Q"=0.0, "Norm  Ampl"=0.0, "z∞ (V)"=0.0+0.0i, "4corners"={"z (-pi/2)"=0.0+0.0i, "z(inf)"=0.0+0.0i, "z (pi/2)"=0.0+0.0i, "z center"=0.0+0.0i, "z(0)"=0.0+0.0i, "radius"=0.0}}, "timestamp(min)"=1730.433333337307, "timestamp"=timestamp(3493831647 s since 1904-01-01), "Magn Field(T)"=0.0}, {"temperature"=32.907, "lorentzian"={"A (VHz)"=0.0, "ω (Hz)"=0.0, "Γ (Hz)"=0.0, "φ (rad)"=0.0, "Q"=0.0, "Norm  Ampl"=0.0, "z∞ (V)"=0.0+0.0i, "4corners"={"z (-pi/2)"=0.0+0.0i, "z(inf)"=0.0+0.0i, "z (pi/2)"=0.0+0.0i, "z center"=0.0+0.0i, "z(0)"=0.0+0.0i, "radius"=0.0}}, "timestamp(min)"=1731.75, "timestamp"=timestamp(3493831726 s since 1904-01-01), "Magn Field(T)"=0.0}, {"temperature"=32.817, "lorentzian"={"A (VHz)"=0.0, "ω (Hz)"=0.0, "Γ (Hz)"=0.0, "φ (rad)"=0.0, "Q"=0.0, "Norm  Ampl"=0.0, "z∞ (V)"=0.0+0.0i, "4corners"={"z (-pi/2)"=0.0+0.0i, "z(inf)"=0.0+0.0i, "z (pi/2)"=0.0+0.0i, "z center"=0.0+0.0i, "z(0)"=0.0+0.0i, "radius"=0.0}}, "timestamp(min)"=1733.0833333358169, "timestamp"=timestamp(3493831806 s since 1904-01-01), "Magn Field(T)"=0.0}, {"temperature"=32.723, "lorentzian"={"A (VHz)"=0.0, "ω (Hz)"=0.0, "Γ (Hz)"=0.0, "φ (rad)"=0.0, "Q"=0.0, "Norm  Ampl"=0.0, "z∞ (V)"=0.0+0.0i, "4corners"={"z (-pi/2)"=0.0+0.0i, "z(inf)"=0.0+0.0i, "z (pi/2)"=0.0+0.0i, "z center"=0.0+0.0i, "z(0)"=0.0+0.0i, "radius"=0.0}}, "timestamp(min)"=1734.3999999985099, "timestamp"=timestamp(3493831885 s since 1904-01-01), "Magn Field(T)"=0.0}, {"temperature"=32.637, 
